vi "SetPan.vi"(9 "Sensor Position":dbl format="%#_13g", 10 "New Command":bool) -> (2 "Reached Setpoint":bool, 3 "Pan Setpoint":dbl format="%#_13g")   [LabVIEW 2015]
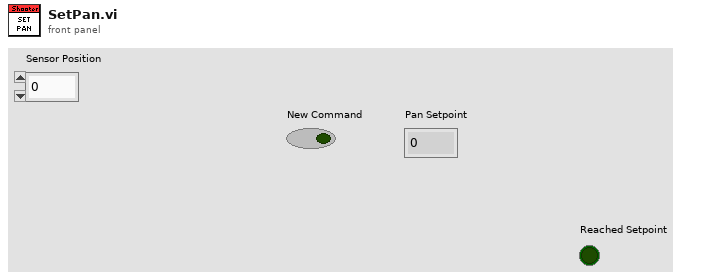
[diagram p1: front panel]
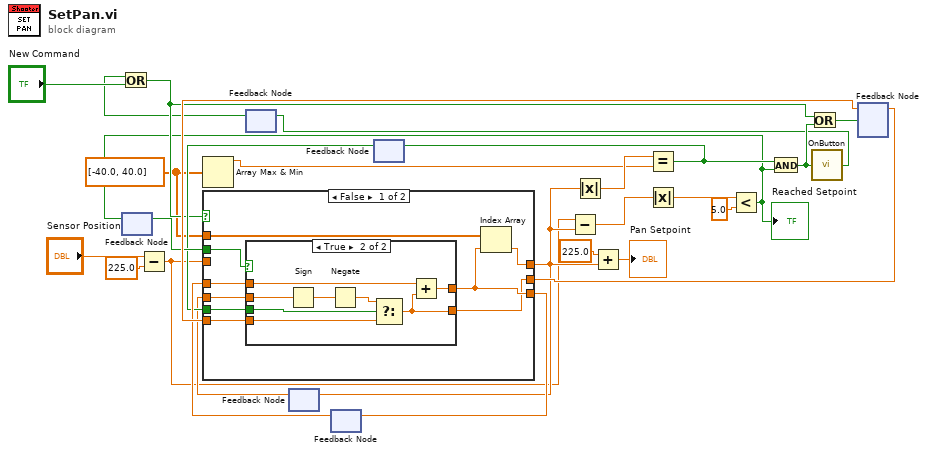
[diagram p0: block diagram]
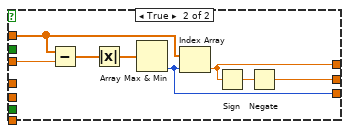
[diagram p3: hidden frame]
diagram:
  w1 = dbl[] [-40.0, 40.0]
  n1 = feedback #1() -> (w18:bool)  [unwired: 1 in]
  n2 = Subtract(x="Sensor Position", y=225.0) -> (x-y=w6:dbl)
  n3 = Array Max & Min(array=w1) -> (max value=w21:dbl)  [unwired: 3 out]
  n4 = feedback #2() -> (w9:bool)  [unwired: 1 in]
  n5 = Or(x=w9, y="New Command") -> (x .or. y?=w11:bool)
  n6 = feedback #3() -> (w12:dbl)  [unwired: 1 in]
  n7 = feedback #4() -> (w17:dbl)  [unwired: 1 in]
  n8 = feedback #5() -> (w16:bool)  [unwired: 1 in]
  n9 = feedback #6() -> (w20:dbl)  [unwired: 1 in]
  n10 = case shown="False" w11 {
    tunnel: w6 -> [_ w54]
    tunnel: w1 -> [w36 w51]
    tunnel: [w35 w50] -> w13
    tunnel: w20 -> [w29 _]
    tunnel: [w28 w47] -> w19
    tunnel: w18 -> [w32 _]
    tunnel: [w33 w48] -> w14
    tunnel: w17 -> [w34 _]
    tunnel: w16 -> [w31 _]
    tunnel: w12 -> [w30 _]
    frame False {
      n11 = case shown="True" w32 {
        tunnel: w29 -> [w37 w45]
        tunnel: [w38 w39] -> w33
        tunnel: w34 -> [w38 w44]
        tunnel: w31 -> [_ w41]
        tunnel: [w37 w46] -> w28
        tunnel: w30 -> [_ w40]
        frame False {
        }
        frame True {
          n12 = Sign(1:w40) -> (0:w43:dbl)
          n13 = Negate(x=w43) -> (-x=w42:dbl)
          n14 = Select(t=w42, s=w41, f=w45) -> (s? t:f=w46:dbl)
          n15 = Add(x=w44, y=w46) -> (x+y=w39:dbl)
        }
      }
      n16 = Index Array(array=w36, index=w33) -> (element=w35:dbl)
    }
    frame True {
      n17 = Subtract(x=w51, y=w54) -> (x-y=w53:dbl[])
      n18 = Absolute Value(x=w53) -> (abs(x)=w52:dbl[])
      n19 = Array Max & Min(array=w52) -> (min index (indices)=w48:i32)  [unwired: 3 out]
      n20 = Index Array(array=w51, index=w48) -> (element=w50:dbl)
      n21 = Sign(1:w50) -> (0:w49:dbl)
      n22 = Negate(x=w49) -> (-x=w47:dbl)
    }
  }
  n23 = feedback-in #3(w13) -> ()
  n24 = feedback-in #4(w14) -> ()
  n25 = Subtract(x=w6, y=w13) -> (x-y=w27:dbl)
  n26 = Absolute Value(x=w13) -> (abs(x)=w22:dbl)
  n27 = Add(x=225.0, y=w13) -> (x+y=→"Pan Setpoint":dbl)
  n28 = Equal?(x=w22, y=w21) -> (x = y?=w15:bool)
  n29 = feedback-in #5(w15) -> ()
  n30 = Absolute Value(x=w27) -> (abs(x)=w26:dbl)
  n31 = Less?(x=w26, y=5.0) -> (x < y?=w2:bool)
  "Reached Setpoint" <- w2
  n32 = feedback-in #1(w2) -> ()
  n33 = And(x=w15, y=w2) -> (x .and. y?=w10:bool)
  n34 = Or(x=w11, y=w10) -> (x .or. y?=w24:bool)
  n35 = call "OnButton.vi"("Button"=w10) -> ("Value"=w8:bool)  [unwired: 1 in]
  n36 = feedback-in #2(w8) -> ()
  n37 = feedback-in #6(w19, w24) -> ()
